vi "feet to encoder ticsk.vi"(11 "Distance in feet wanted":dbl) -> (3 "Encoder Ticks":dbl)   [LabVIEW 2017]
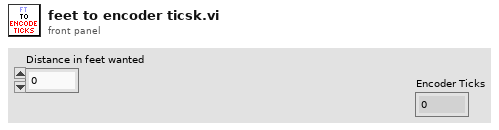
[diagram p1: front panel]
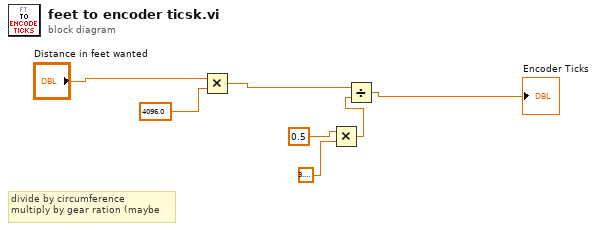
[diagram p0: block diagram]
diagram:
  # "divide by circumference\nmultiply by gear ration (maybe"
  n1 = Multiply(x="Distance in feet wanted", y=4096.0) -> (x*y=w5:dbl)
  n2 = Multiply(x=0.5, y=3.141592653589793) -> (x*y=w2:dbl)
  n3 = Divide(x=w5, y=w2) -> (x/y=→"Encoder Ticks":dbl)
